vi "Error.vi"(8 "error in (no error)":errorcluster, 11 "message queue in":T1) -> (0 "error out":errorcluster)   [LabVIEW 2013]
uses:
  <vilib>/NI/AMC/Message Queue.ctl
  <vilib>/NI/AMC/Message.ctl
  <vilib>/NI/Tools/Keyed Array/KeyedArray.ctl
  <vilib>/NI/AMC/Create Single Message.vi
  <vilib>/NI/AMC/Update Message Routing Info.vi
  <vilib>/NI/AMC/Send Message.vi
  <vilib>/NI/AMC/AMC.lvlib
  <vilib>/NI/Tools/Keyed Array/Tools_KeyedArray.lvlib
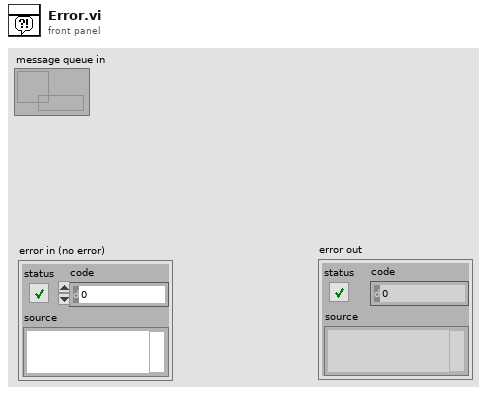
[diagram p1: front panel]
types:
  T1 = typedef "AMC.lvlib/Message Queue.ctl" = refnum<queue>
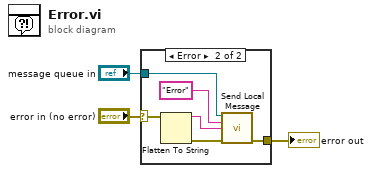
[diagram p0: block diagram]
diagram:
  n1 = case shown="Error" "error in (no error)" {
    selector: "error in (no error)" -> [_ w5]
    tunnel: [_ w9] -> w3
    tunnel: "message queue in" -> [_ w8]
    frame No Error {
    }
    frame Error {
      n2 = Flatten To String(anything=w5) -> (data string=w4:string, error out=w6:errorcluster)  [unwired: 3 in, 1 out]
      n3 = call <vilib>:"Send Local Message.vi"("message queue in"=w8, "message name"="Error", "message value"=w4, "error in"=w6) -> ("error out"=w9:errorcluster)  [unwired: 9 in, 2 out]
    }
  }
  "error out" <- w3
